vi "Initialize.vi"(8 "error in":errorcluster, 10 "Device":string) -> (0 "error out":errorcluster, 3 "Thermocouple out":refnum<class "Thermocouple.lvclass">)   [LabVIEW 2018, in "Thermocouple.lvlib" / "Thermocouple.lvclass"]
uses:
  Thermocouple.lvclass
  Thermocouple.lvclass/Thermocouple.ctl
  PPLs/Configuration/Configuration.lvlibp/Configuration.lvclass
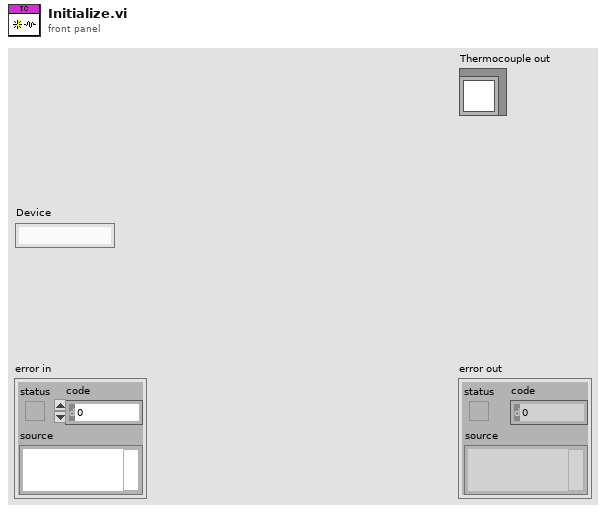
[diagram p1: front panel]
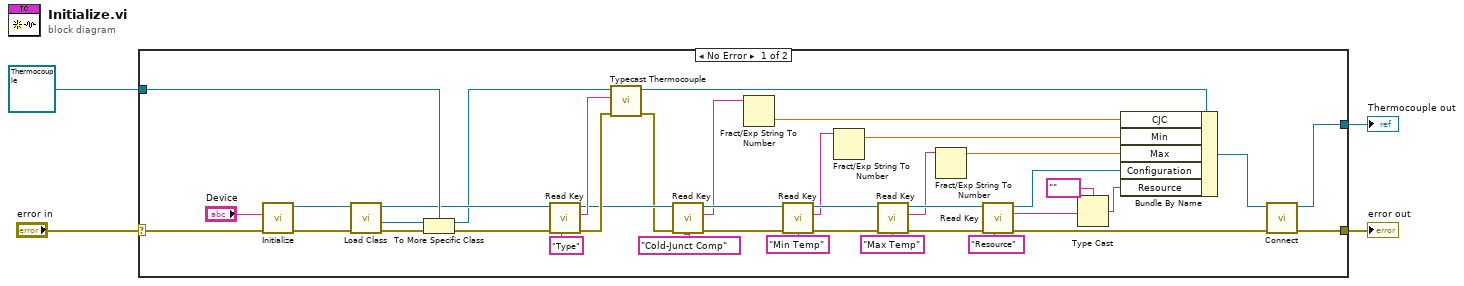
[diagram p0: block diagram]
diagram:
  n1 = case shown="No Error" "error in" {
    selector: "error in" -> [w43 w46]
    tunnel: [w32 w46] -> w3
    tunnel: [w34 w45] -> w1
    tunnel: refnum<class "Thermocouple.lvclass"> refnum ("Thermocouple in") -> [w35 w45]
    frame No Error {
      n2 = call "Initialize.vi"("error in"=w43, "Device"="Device") -> ("error out"=w41:errorcluster, "Configuration out"=w42:refnum<class "Configuration.lvclass">)  [unwired: 8 in]
      n3 = call "Load Class.vi"("error in"=w41, "Configuration in"=w42) -> ("error out"=w40:errorcluster, "Class out"=w39:refnum<class>, "Configuration out"=w27:refnum<class "Configuration.lvclass">)  [unwired: 7 in]
      n4 = To More Specific Class(target class=w35, reference=w39, error in=w40) -> (specific class reference=w25:refnum<class "Thermocouple.lvclass">, error out=w28:errorcluster)
      n5 = call "Read Key.vi"("Key:"="Type", "error in"=w28, "Configuration in"=w27) -> ("error out"=w23:errorcluster, "Value"=w24:string, "Configuration out"=w20:refnum<class "Configuration.lvclass">)  [unwired: 6 in]
      n6 = call "Typecast Thermocouple.vi"("error in (no error)"=w23, "Thermocouple Type"=w24, "Thermocouple in"=w25) -> ("error out"=w17:errorcluster, "Thermocouple out"=w22:refnum<class "Thermocouple.lvclass">)  [unwired: 7 in]
      n7 = call "Read Key.vi"("Key:"="Cold-Junct Comp", "error in"=w17, "Configuration in"=w20) -> ("error out"=w13:errorcluster, "Value"=w10:string, "Configuration out"=w16:refnum<class "Configuration.lvclass">)  [unwired: 6 in]
      n8 = Fract/Exp String To Number(string=w10) -> (number=w9:dbl)  [unwired: 3 in, 1 out]
      n9 = call "Read Key.vi"("Key:"="Min Temp", "error in"=w13, "Configuration in"=w16) -> ("error out"=w12:errorcluster, "Value"=w8:string, "Configuration out"=w15:refnum<class "Configuration.lvclass">)  [unwired: 6 in]
      n10 = Fract/Exp String To Number(string=w8) -> (number=w7:dbl)  [unwired: 3 in, 1 out]
      n11 = call "Read Key.vi"("Key:"="Max Temp", "error in"=w12, "Configuration in"=w15) -> ("error out"=w11:errorcluster, "Value"=w6:string, "Configuration out"=w14:refnum<class "Configuration.lvclass">)  [unwired: 6 in]
      n12 = Fract/Exp String To Number(string=w6) -> (number=w5:dbl)  [unwired: 3 in, 1 out]
      n13 = call "Read Key.vi"("Key:"="Resource", "error in"=w11, "Configuration in"=w14) -> ("error out"=w33:errorcluster, "Value"=w37:string, "Configuration out"=w38:refnum<class "Configuration.lvclass">)  [unwired: 6 in]
      n14 = Type Cast(type=tag "" ("Resource"), x=w37) -> (*(type *) &x=w30:tag)
      n15 = Bundle By Name(cluster=w22, "CJC"=w9, "Min"=w7, "Max"=w5, "Configuration"=w38, "Resource"=w30) -> (w36:refnum<class "Thermocouple.lvclass">)
      n16 = call-dynamic "Connect.vi"("error in (no error)"=w33, "Thermocouple in"=w36) -> ("error out"=w32:errorcluster, "Thermocouple out"=w34:refnum<class "Thermocouple.lvclass">)  [unwired: 8 in]
    }
    frame Error {
    }
  }
  "error out" <- w3
  "Thermocouple out" <- w1
